vi "LEBITVacuum.ParseSafetyArray.vi"(1 "Safety Array":string[][](array[string])) -> (15 "CloseSafetyOverwritePLC":string[](array[string]), 16 "OpenSafetyOverwritePLC":string[](array[string]), 17 "CloseSafetyOverwritePLCServiceID":i32[](array[numeric]), 18 "OpenSafetyOverwritePLCServiceID":i32[](array[numeric]))   [LabVIEW 2014, in "LEBITVacuum.lvlib"]
uses:
  LEBITVacuum.lvlib
panel:
  out "nickname":string[](array[string])
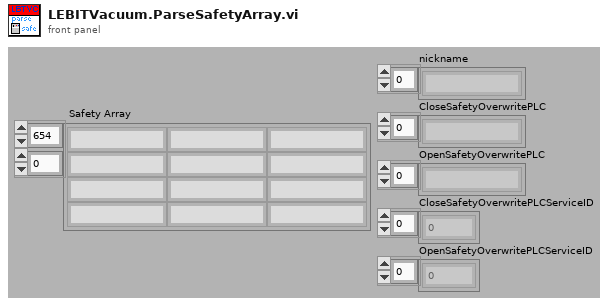
[diagram p1: front panel]
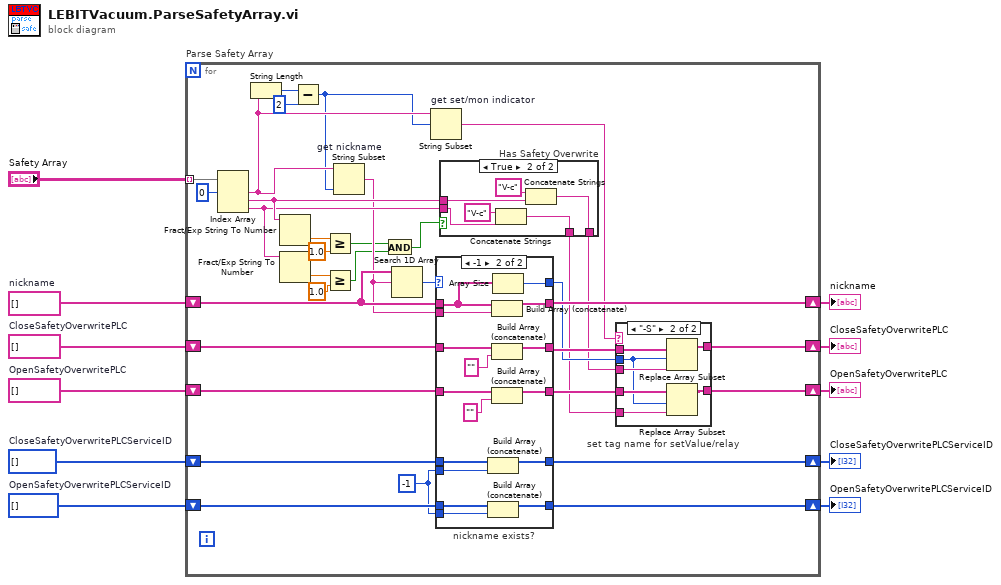
[diagram p0: block diagram]
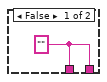
[diagram p2: hidden frame]
diagram:
  w3 = i32[] []  # OpenSafetyOverwritePLCServiceID
  w4 = i32[] []  # CloseSafetyOverwritePLCServiceID
  w8 = string[] []  # OpenSafetyOverwritePLC
  w9 = string[] []  # CloseSafetyOverwritePLC
  w11 = string[] []  # nickname
  n1 = for "Parse Safety Array" {
    tunnel: "Safety Array" -> [w45] mode=indexing
    shift-right: [w35] -> w7
    shift-left: w11 -> [w38]
    shift-right: [w34] -> w5
    shift-left: w8 -> [w31]
    shift-right: [w30] -> w6
    shift-left: w9 -> [w32]
    shift-right: [w12] -> w2
    shift-left: w4 -> [w16]
    shift-right: [w14] -> w1
    shift-left: w3 -> [w15]
    w13 = -1
    n2 = Index Array(array=w45, index #1=0 ("index")) -> (element #1=w41:string, element #2=w26:string, element #3=w25:string)  [unwired: 2 in]
    n3 = String Length(string=w41) -> (length=w43:i32)
    n4 = Fract/Exp String To Number(string=w26) -> (number=w17:dbl)  [unwired: 3 in, 1 out]
    n5 = Fract/Exp String To Number(string=w25) -> (number=w19:dbl)  [unwired: 3 in, 1 out]
    n6 = Subtract(x=w43, y=2) -> (x-y=w40:i32)
    n7 = Greater Or Equal?(x=w17, y=1.0 ("x")) -> (x >= y?=w22:bool)
    n8 = Greater Or Equal?(x=w19, y=1.0 ("x")) -> (x >= y?=w23:bool)
    n9 = String Subset "get nickname"(string=w41, length (rest)=w40) -> (substring=w24:string)  [unwired: 1 in]
    n10 = And(x=w22, y=w23) -> (x .and. y?=w21:bool)
    n11 = Search 1D Array(1D array=w38, element=w24) -> (index of element=w39:i32)  [unwired: 1 in]
    n12 = String Subset "get set/mon indicator"(string=w41, offset (0)=w40) -> (substring=w33:string)  [unwired: 1 in]
    n13 = case "nickname exists?" shown="-1" w39 {
      selector: w39 -> [w56 _]
      tunnel: w38 -> [w58 w69]
      tunnel: w24 -> [_ w74]
      tunnel: [w58 w73] -> w35
      tunnel: w31 -> [w57 w72]
      tunnel: [w55 w71] -> w37
      tunnel: [w57 w70] -> w36
      tunnel: [w56 w68] -> w29
      tunnel: w32 -> [w55 w67]
      tunnel: w16 -> [w54 w64]
      tunnel: [w54 w63] -> w12
      tunnel: w15 -> [w53 w60]
      tunnel: [w53 w62] -> w14
      tunnel: w13 -> [_ w61]
      tunnel: w13 -> [_ w59]
      frame 0, Default {
      }
      frame -1 {
        n14 = Build Array (concatenate)(w64, w61) -> (w63:i32[])
        n15 = Build Array (concatenate)(w60, w59) -> (w62:i32[])
        n16 = Build Array (concatenate)(w69, w74) -> (w73:string[])
        n17 = Build Array (concatenate)(w67, "") -> (w71:string[])
        n18 = Build Array (concatenate)(w72, "") -> (w70:string[])
        n19 = Array Size(array=w69) -> (size(s)=w68:i32)
      }
    }
    n20 = case "Has Safety Overwrite" shown="True" w21 {
      tunnel: [w46 w50] -> w28
      tunnel: [w46 w49] -> w27
      tunnel: w26 -> [_ w48]
      tunnel: w25 -> [_ w47]
      frame False {
        w46 = ""
      }
      frame True {
        n21 = Concatenate Strings("V-c" ("string"), w47) -> (w50:string)
        n22 = Concatenate Strings("V-c" ("string"), w48) -> (w49:string)
      }
    }
    n23 = case "set tag name for setValue/relay" shown="\"-S\"" w33 {
      tunnel: w37 -> [w76 w83]
      tunnel: w29 -> [_ w77]
      tunnel: w27 -> [_ w82]
      tunnel: w36 -> [w75 w79]
      tunnel: w28 -> [_ w78]
      tunnel: [w76 w81] -> w30
      tunnel: [w75 w80] -> w34
      frame Default {
      }
      frame "-S" {
        n24 = Replace Array Subset(array=w83, new element=w82, index=w77) -> (w81:string[])
        n25 = Replace Array Subset(array=w79, new element=w78, index=w77) -> (w80:string[])
      }
    }
  }
  "nickname" <- w7
  "CloseSafetyOverwritePLC" <- w6
  "OpenSafetyOverwritePLC" <- w5
  "CloseSafetyOverwritePLCServiceID" <- w2
  "OpenSafetyOverwritePLCServiceID" <- w1
